vi "Open SV.vi"(6 "PC Name":string, 8 "error in (no error)":errorcluster, 9 "SV Name":string, 10 "SV":refnum<k21>, 11 "AEgIS Shared Variables in":refnum<class "Circus Shared Variables.lvclass">) -> (0 "error out":errorcluster, 3 "AEgIS Shared Variables out":refnum<class "Circus Shared Variables.lvclass">)   [LabVIEW 2026, in "TALOS.lvlib" / "Classes.lvlib" / "Circus Shared Variables.lvclass"]
doc: "Use this VI to to open the connection to a Shared Variable. If the Var Ref is given in input, it ignores the name and use that; otherwise, it looks for a variable with the name given and uses the FIRST FOUND.\nIf PC name is wired as input, the SV will be looked on that specific pc: useful to increases search speed, if the location of the SV is known a priori."
uses:
  Circus Shared Variables.lvclass
  Circus Shared Variables.lvclass/Circus Shared Variables.ctl
  Ancestor/Ancestor/Ancestor.lvclass/Ancestor.ctl
  FGV/Error Memory/Get Error Description.vi
  Support VIs/Get PC name.vi
  Ancestor/Ancestor/Read ID.vi
  Support VIs/Get Class Name.vi
  <vilib>/Utility/error.llb/Clear Errors.vi
  FGV/Error Memory/Error Memory Core.vi
  <vilib>/AdvancedString/Delimited String to 1D String Array.vi
  <vilib>/AdvancedString/Delimited String to 1D String Array (string).vi
  Support VIs/Circus Root Path.vi
  FGV/Error Memory/Error Crt Lvl checker.vi
  FGV/Error Memory/Error Memory Core.vi/40c8088d-b597-4017-91af-faa98e00292e.vi
  FGV/Error Memory/Error Memory Core.vi/d4a3ab98-063c-4e44-b43d-fbdcfe6c2be2.vi
  Support VIs/Global Constants.vi
  Support VIs/Global Memory.vi
  <vilib>/Utility/LVClass/Get LV Class Name.vi
  Support VIs/Is in Packed Library.vi
  Support VIs/TALOS Root path.vi
  Support VIs/Read CSV worksheet.vi
  <vilib>/Utility/error.llb/General Error Handler.vi
  Support VIs/Error Log.vi
  <vilib>/Utility/config.llb/Open Config Data.vi
  <vilib>/Utility/config.llb/Get Section Names.vi
  <vilib>/Utility/config.llb/Get Key Names.vi
  <vilib>/Utility/config.llb/Read Key.vi
  <vilib>/Utility/config.llb/Read Key (String).vi
  <vilib>/Utility/config.llb/Close Config Data.vi
  Ancestor/Ancestor/Ancestor.lvclass
  <vilib>/Comparison/Equal/Equal Functor/Equal Functor.lvclass
  TALOS.lvlib
  <resource>/objmgr/ni.var.rc
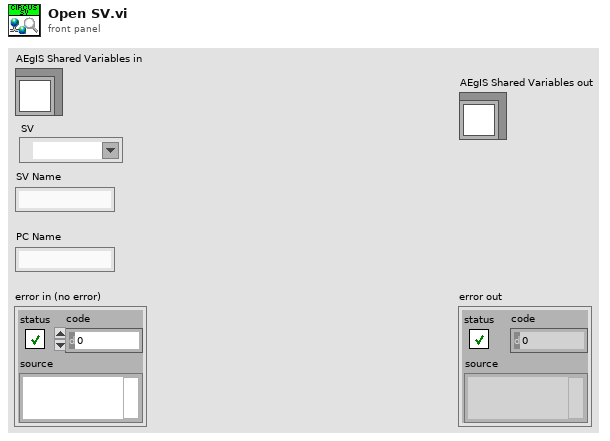
[diagram p1: front panel]
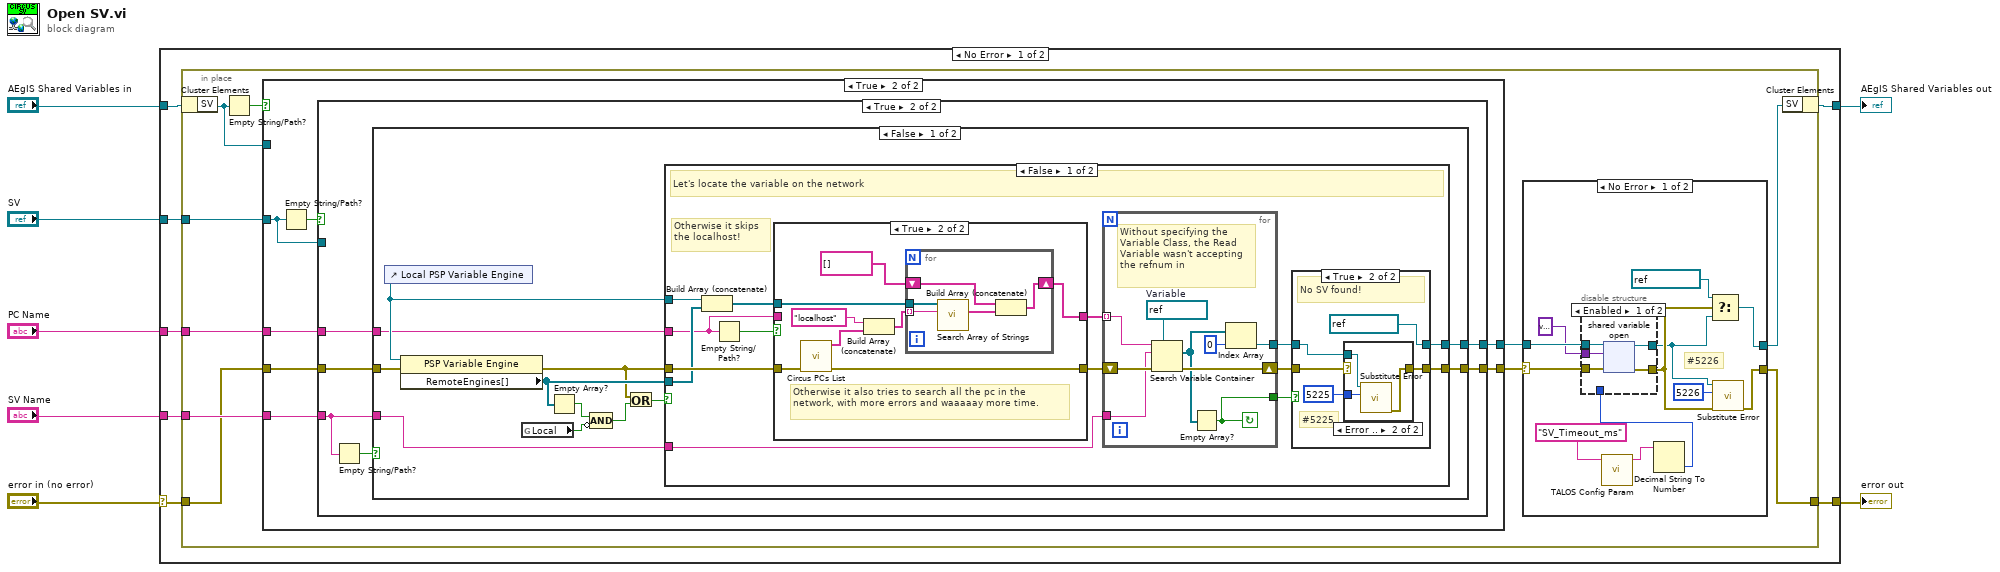
[diagram p0: block diagram]
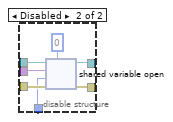
[diagram p2: hidden frame]
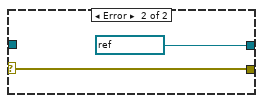
[diagram p3: hidden frame]
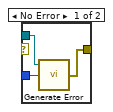
[diagram p7: hidden frame]
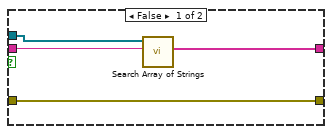
[diagram p8: hidden frame]
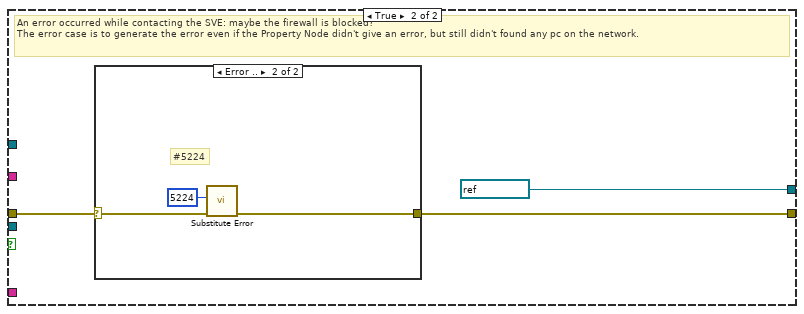
[diagram p9: hidden frame]
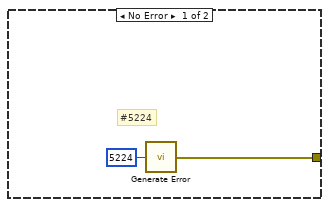
[diagram p10: hidden frame]
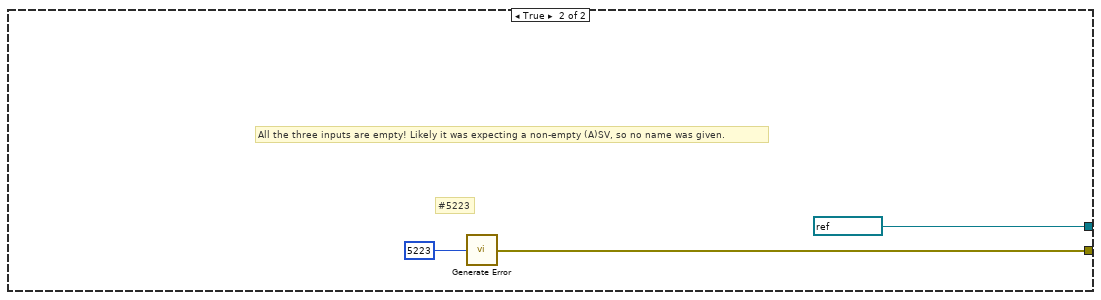
[diagram p11: hidden frame]
diagram:
  n1 = case shown="No Error" "error in (no error)" {
    selector: "error in (no error)" -> [w12 w145]
    tunnel: [w9 w145] -> w6
    tunnel: [w10 w144] -> w5
    tunnel: "AEgIS Shared Variables in" -> [w11 w144]
    tunnel: "SV" -> [w14 _]
    tunnel: "SV Name" -> [w13 _]
    tunnel: "PC Name" -> [w8 _]
    frame No Error {
      n2 = in-place {
        in-place-border: w14 -> [w24]
        in-place-border: w13 -> [w23]
        in-place-border: w12 -> [w22]
        in-place-border: [w18] -> w9
        in-place-border: w8 -> [w17]
        n3 = in-place-cluster #1(w11) -> ("SV"=w16:refnum<k21>)
        n4 = Empty String/Path?(string/path=w16) -> (empty?=w15:bool)
        n5 = case shown="True" w15 {
          tunnel: w24 -> [_ w59]
          tunnel: w23 -> [_ w58]
          tunnel: w22 -> [w52 w57]
          tunnel: [w51 w56] -> w21
          tunnel: [w52 w55] -> w19
          tunnel: w17 -> [_ w54]
          tunnel: w16 -> [w51 _]
          frame False {
          }
          frame True {
            n6 = Empty String/Path?(string/path=w59) -> (empty?=w53:bool)
            n7 = case shown="True" w53 {
              tunnel: w57 -> [w60 w67]
              tunnel: w58 -> [_ w62]
              tunnel: [w61 w64] -> w56
              tunnel: [w60 w66] -> w55
              tunnel: w59 -> [w61 _]
              tunnel: w54 -> [_ w65]
              frame False {
              }
              frame True {
                n8 = Empty String/Path?(string/path=w62) -> (empty?=w63:bool)
                n9 = case shown="False" w63 {
                  tunnel: w67 -> [w78 _]
                  tunnel: [w77 w142] -> w66
                  tunnel: w62 -> [w76 _]
                  tunnel: w65 -> [w75 _]
                  tunnel: [w74 refnum<k21> "1nv4l1d" ("SV")] -> w64
                  frame False {
                    n10 = control-ref of="Local PSP Variable Engine"() -> (w79:refnum<k21>)
                    n11 = property class="PSP Variable Engine"(reference=w79, error in=w78) -> (error out=w68:errorcluster, "RemoteEngines[]"=w73:refnum<k21>[])  [unwired: 1 out]
                    n12 = global read "Global Constants.vi" "Local"() -> (w72:bool)
                    n13 = Empty Array?(array=w73) -> (empty?=w71:bool)
                    n14 = Compound Arithmetic op=AND(w71, invert w72) -> (w69:bool)
                    n15 = Or(x=w68, y=w69) -> (x .or. y?=w70:bool)
                    n16 = case shown="False" w70 {
                      tunnel: w79 -> [w91 _]
                      tunnel: w68 -> [w90 w134]
                      tunnel: w73 -> [w88 _]
                      tunnel: [w80 w133] -> w77
                      tunnel: w76 -> [w87 _]
                      tunnel: w75 -> [w85 _]
                      tunnel: [w81 refnum<k21> "1nv4l1d" ("SV")] -> w74
                      frame False {
                        # "Otherwise it skips the localhost!"
                        # "Let's locate the variable on the network"
                        n17 = Build Array (concatenate)(w91, w88) -> (w93:refnum<k21>[])
                        n18 = Empty String/Path?(string/path=w85) -> (empty?=w86:bool)
                        n19 = case shown="True" w86 {
                          tunnel: w93 -> [w109 w118]
                          tunnel: [w107 w117] -> w92
                          tunnel: w90 -> [w110 w115]
                          tunnel: [w110 w114] -> w89
                          tunnel: w85 -> [w108 _]
                          frame False {
                            n20 = call "Search Array of Strings.vi"("search string"=w108, "Search array"=w109) -> ("found elements"=w107:string[])  [unwired: 8 in, 1 out]
                          }
                          frame True {
                            # "Otherwise it also tries to search all the pc in the network, with more errors and waaaaay more time."
                            n21 = call "Circus PCs List.vi"("error in (no error)"=w115) -> ("error out"=w114:errorcluster, "PC List out"=w112:string[])  [unwired: 9 in]
                            n22 = Build Array (concatenate)("localhost", w112) -> (w113:string[])
                            n23 = for {
                              tunnel: w118 -> [w123]
                              tunnel: w113 -> [w120] mode=indexing
                              shift-right: [w122] -> w117
                              shift-left: string[] [] -> [w119]
                              n24 = call "Search Array of Strings.vi"("search string"=w120, "Search array"=w123) -> ("found elements"=w121:string[])  [unwired: 8 in, 1 out]
                              n25 = Build Array (concatenate)(w119, w121) -> (w122:string[])
                            }
                          }
                        }
                        n26 = for {
                          shift-right: [w131] -> w84
                          shift-left: w89 -> [w130]
                          tunnel: w92 -> [w129] mode=indexing
                          tunnel: w87 -> [w128]
                          tunnel: [w125] -> w83
                          tunnel: [w124] -> w82
                          stop <- w124 continue-if-true
                          w132 = refnum<k21> refnum  # Variable
                          # "Without specifying the Variable Class, the Read Variable wasn't accepting the refnum in"
                          n27 = Search Variable Container(7:w132, 8:w130, 10:w128, 11:w129) -> (0:w131:errorcluster, 2:w127:refnum<k21>[])  [unwired: 2 in, 1 out]
                          n28 = Empty Array?(array=w127) -> (empty?=w124:bool)
                          n29 = Index Array(array=w127, index=0) -> (element=w125:refnum<k21>)
                        }
                        n30 = case shown="True" w82 {
                          tunnel: w84 -> [w94 w99]
                          tunnel: w83 -> [w95 w96]
                          tunnel: [w95 refnum<k21> "1nv4l1d" ("SV")] -> w81
                          tunnel: [w94 w98] -> w80
                          frame False {
                            # "At least one SV was found."
                          }
                          frame True {
                            # "#5225"
                            # "No SV found!"
                            n31 = case shown="Error .." w99 {
                              tunnel: [w103 w105] -> w98
                              tunnel: 5225 ("index") -> [w102 w106]
                              tunnel: w96 -> [w101 w104]
                              frame No Error {
                                n32 = call "Generate Error.vi"("Optional String"=w101, "Error Code"=w102) -> ("error out"=w103:errorcluster)  [unwired: 5 in]
                              }
                              frame Error {
                                n33 = call "Substitute Error.vi"("Error Code"=w106, "Optional String"=w104) -> ("error out"=w105:errorcluster)  [unwired: 9 in]
                              }
                            }
                          }
                        }
                      }
                      frame True {
                        # "An error occurred while contacting the SVE: maybe the firewall is blocked?\nThe error case is to generate the error even if the Property Node didn't give an error, but still didn't found any pc on the network."
                        n34 = case shown="Error .." w134 {
                          selector: w134 -> [_ w140]
                          tunnel: [w137 w138] -> w133
                          frame No Error {
                            # "#5224"
                            n35 = call "Generate Error.vi"("Error Code"=5224) -> ("error out"=w137:errorcluster)  [unwired: 6 in]
                          }
                          frame Error {
                            # "#5224"
                            n36 = call "Substitute Error.vi"("error in (no error)"=w140, "Error Code"=5224) -> ("error out"=w138:errorcluster)  [unwired: 9 in]
                          }
                        }
                      }
                    }
                  }
                  frame True {
                    # "#5223"
                    # "All the three inputs are empty! Likely it was expecting a non-empty (A)SV, so no name was given."
                    n37 = call "Generate Error.vi"("Error Code"=5223) -> ("error out"=w142:errorcluster)  [unwired: 6 in]
                  }
                }
              }
            }
          }
        }
        n38 = case shown="No Error" w19 {
          selector: w19 -> [w35 w50]
          tunnel: w21 -> [w36 _]
          tunnel: [w28 refnum<k21> "1nv4l1d" ("SV")] -> w20
          tunnel: [w30 w50] -> w18
          frame No Error {
            # "#5226"
            n39 = call "TALOS Config Param.vi"("Parameter Name"="SV_Timeout_ms") -> ("Output"=w33:string)  [unwired: 9 in, 1 out]
            n40 = Decimal String To Number(string=w33) -> (number=w31:i32)  [unwired: 2 in, 1 out]
            n41 = disable-structure shown="Enabled" {
              disable-tunnel: w36 -> [w41 w48]
              disable-tunnel: [w40 w47] -> w25
              disable-tunnel: w35 -> [w39 w46]
              disable-tunnel: [w38 w45] -> w29
              disable-tunnel: variant ("data type") -> [w37 w44]
              disable-tunnel: w31 -> [_ w42]
              frame Enabled {
                n42 = shared-variable-open(w41, w39, w37) -> (w40:refnum<k21>, w38:errorcluster)
              }
              frame Disabled {
                n43 = shared-variable-open(w48, w46, w44, w42, u32 0 ("buffer size in elements")) -> (w47:refnum<k21>, w45:errorcluster)
              }
            }
            n44 = Select(t=refnum<k21> "1nv4l1d" ("SV"), s=w29, f=w25) -> (s? t:f=w28:refnum<k21>)
            n45 = call "Substitute Error.vi"("error in (no error)"=w29, "Error Code"=5226, "Optional String"=w25) -> ("error out"=w30:errorcluster)  [unwired: 8 in]
          }
          frame Error {
          }
        }
        n46 = in-place-cluster #1("SV"=w20) -> (w10:refnum<class "Circus Shared Variables.lvclass">)
      }
    }
    frame Error {
    }
  }
  "error out" <- w6
  "AEgIS Shared Variables out" <- w5
